vi "CheckVI.vi"(8 "error in (no error)":errorcluster, 11 "VI Refnum":refnum<vi>) -> (0 "error out":errorcluster, 1 "Output/Failure":string, 2 "CLI Process Return Code":i32, 3 "dup VI Refnum":refnum<vi>, 4 "Reject?":bool)   [LabVIEW 2014, in "BuildSecurity.lvlib"]
doc: "Checks the VI for any blacklisted items. If any items are found, <b>Reject?</b> will return <b>TRUE</b>."
uses:
  BuildSecurity.lvlib
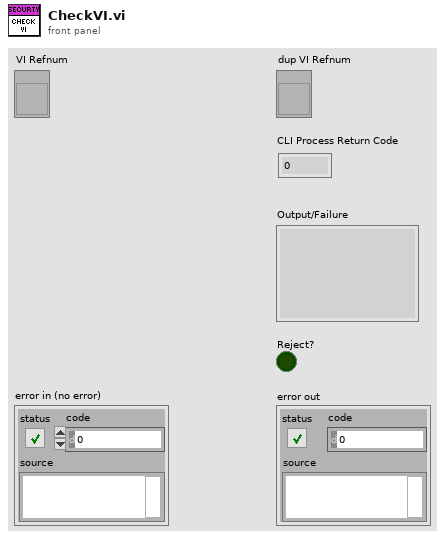
[diagram p1: front panel]
types:
  T1 = typedef "BuildSecurity.lvlib/BlacklistClassInfo.ctl" = cluster{"Class":string, "Items":string[]}
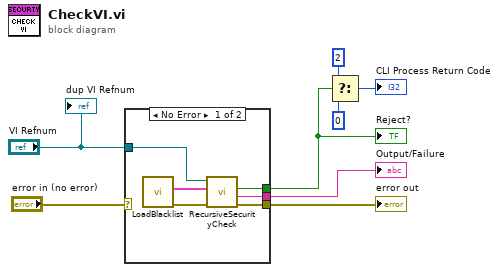
[diagram p0: block diagram]
diagram:
  n1 = case shown="No Error" "error in (no error)" {
    selector: "error in (no error)" -> [_ w15]
    tunnel: "VI Refnum" -> [w12 _]
    tunnel: [w11 w15] -> w6
    tunnel: [w10 _] -> w3
    tunnel: [w9 _] -> w5
    frame No Error {
      n2 = call "LoadBlacklist.vi"() -> ("error out"=w13:errorcluster, "Blacklist"=w14:T1[])  [unwired: 10 in]
      n3 = call "RecursiveSecurityCheck.vi"("error in (no error)"=w13, "Blacklist"=w14, "VI Refnum"=w12) -> ("error out"=w11:errorcluster, "Output/Failure"=w9:string, "Reject?"=w10:bool)  [unwired: 5 in, 1 out]
    }
    frame Error {
    }
  }
  "Reject?" <- w3
  "error out" <- w6
  "Output/Failure" <- w5
  n4 = Select(t=2 ("CLI Process Return Code"), s=w3, f=0 ("CLI Process Return Code")) -> (s? t:f=→"CLI Process Return Code":i32)
  "dup VI Refnum" <- "VI Refnum"
